vi "Synthesize Envelope.vi"(0 "MRN in":refnum<class "Moving Ripple Noise.lvclass">, 7 "Fs (Hz)":dbl, 9 "Npts":i32, 11 "error in (no error)":errorcluster) -> (4 "MRN out":refnum<class "Moving Ripple Noise.lvclass">, 8 "Envelope":dbl[][](array[numeric]), 15 "error out":errorcluster)   [LabVIEW 2015, in "Moving Ripple Noise.lvclass"]
uses:
  Moving Ripple Noise.lvclass
  Moving Ripple Noise.lvclass/Moving Ripple Noise.ctl
  Utility VIs/Math VIs/LinSpace (x0-dx-npts).vi
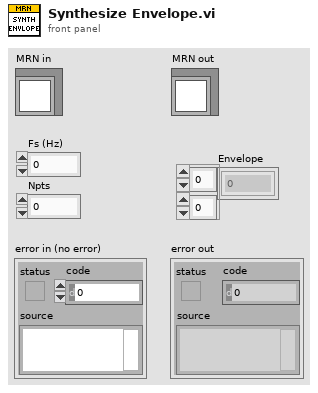
[diagram p1: front panel]
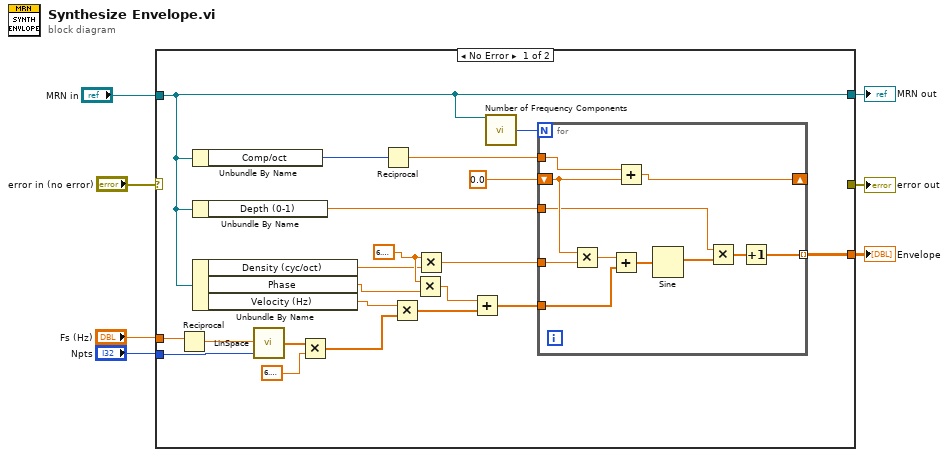
[diagram p0: block diagram]
diagram:
  n1 = case shown="No Error" "error in (no error)" {
    selector: "error in (no error)" -> [_ w41]
    tunnel: "Fs (Hz)" -> [w12 _]
    tunnel: "Npts" -> [w11 _]
    tunnel: "MRN in" -> [w9 w40]
    tunnel: [_ w41] -> w1
    tunnel: [w9 w40] -> w4
    tunnel: [w10 _] -> w3
    frame No Error {
      w18 = 6.283185307179586
      n2 = Reciprocal(x=w12) -> (1/x=w28:dbl)
      n3 = Unbundle By Name(w9) -> ("Comp/oct"=w24:i32)
      n4 = Unbundle By Name(w9) -> ("Depth (0-1)"=w26:dbl)
      n5 = Unbundle By Name(w9) -> ("Density (cyc/oct)"=w16:dbl, "Phase"=w17:dbl, "Velocity (Hz)"=w15:dbl)
      n6 = call-poly "LinSpace.vi"("npts"=w11, "dx"=w28) -> ("Array"=w13:dbl[])  [unwired: 2 in, 1 out]
      n7 = Multiply(x=w13, y=6.283185307179586) -> (x*y=w27:dbl[])
      n8 = Reciprocal(x=w24) -> (1/x=w25:dbl)
      n9 = Multiply(x=w15, y=w27) -> (x*y=w21:dbl[])
      n10 = Multiply(x=w18, y=w17) -> (x*y=w23:dbl)
      n11 = Multiply(x=w18, y=w16) -> (x*y=w19:dbl)
      n12 = Add(x=w23, y=w21) -> (x+y=w22:dbl[])
      n13 = call "Number of Frequency Components.vi"("MRN in"=w9) -> ("Nfreq"=w8:i32)  [unwired: 12 in, 2 out]
      n14 = for {
        N: w8 -> [_]
        tunnel: w19 -> [w39]
        shift-right: [w33] -> _
        shift-left: 0.0 -> [w35]
        tunnel: w22 -> [w37]
        tunnel: w25 -> [w34]
        tunnel: w26 -> [w31]
        tunnel: [w29] -> w10 mode=indexing
        n15 = Multiply(x=w35, y=w39) -> (x*y=w38:dbl)
        n16 = Add(x=w38, y=w37) -> (x+y=w36:dbl[])
        n17 = Add(x=w34, y=w35) -> (x+y=w33:dbl)
        n18 = Sine(x=w36) -> (sin(x)=w32:dbl[])
        n19 = Multiply(x=w31, y=w32) -> (x*y=w30:dbl[])
        n20 = Increment(x=w30) -> (x+1=w29:dbl[])
      }
    }
    frame Error {
    }
  }
  "error out" <- w1
  "MRN out" <- w4
  "Envelope" <- w3
